vi "initialize lcr.vi"() -> (3 "lcr out":refnum<visa-resource-name>)   [LabVIEW 2018]
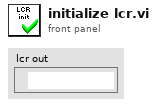
[diagram p1: front panel]
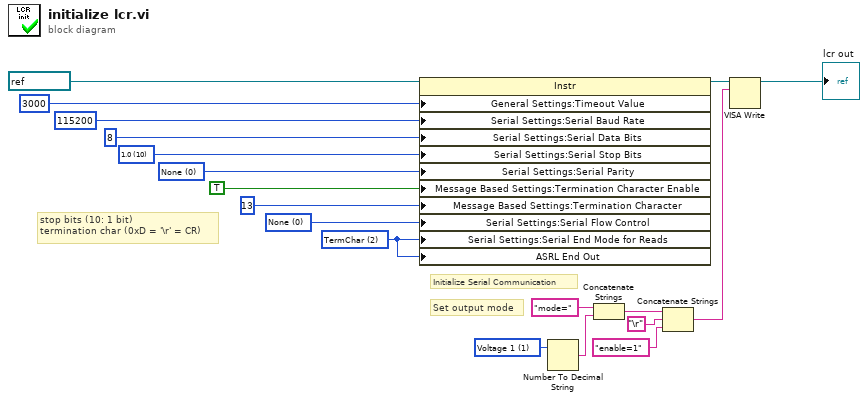
[diagram p0: block diagram]
diagram:
  w11 = u16 1 items=["Modulate", "Voltage 1", "Voltage 2"] ("Output Mode")
  w12 = u16 2 items=["None", "LastBit", "TermChar"] ("Serial Settings:Serial End Mode for Reads")
  w16 = u16 0 items=["None", "XON/XOFF", "RTS/CTS", "XON/XOFF & RTS/CTS", "DTR/DSR", "XON/XOFF & DTR/DSR"] ("flow control (0:none)")
  w14 = u16 0 items=["None", "Odd", "Even", "Mark", "Space"] ("Serial Settings:Parity")
  w18 = u16 10 items=["1.0"=10, "1.5"=15, "2.0"=20]
  # "stop bits (10: 1 bit)\ntermination char (0xD = '\\r' = CR)"
  # "Set output mode"
  # "Initialize Serial Communication"
  n1 = property class="Instr"(reference=refnum<visa-resource-name> "LCC25" ("VISA resource name"), "General Settings:Timeout Value"=u32 3000 ("timeout (10sec)"), "Serial Settings:Serial Baud Rate"=u32 115200 ("baud rate (9600)115200"), "Serial Settings:Serial Data Bits"=u16 8 ("data bits (8)"), "Serial Settings:Serial Stop Bits"=w18, "Serial Settings:Serial Parity"=w14, "Message Based Settings:Termination Character Enable"=TRUE ("Enable Termination\nChar (T)"), "Message Based Settings:Termination Character"=u8 13, "Serial Settings:Serial Flow Control"=w16, "Serial Settings:Serial End Mode for Reads"=w12, "ASRL End Out"=w12) -> (reference out=w3:refnum<visa-resource-name>)  [unwired: 1 in, 1 out]
  n2 = Number To Decimal String(number=w11) -> (decimal integer string=w10:string)  [unwired: 1 in]
  n3 = Concatenate Strings("mode=" ("string"), w10) -> (w5:string)
  n4 = Concatenate Strings(w5, "\r", "enable=1" ("write buffer")) -> (w4:string)
  n5 = VISA Write(VISA resource name=w3, write buffer=w4) -> (VISA resource name out=→"lcr out":refnum<visa-resource-name>)  [unwired: 1 in, 2 out]
